vi "Simple Add.vi"() -> ()   [LabVIEW 2018]
panel:
  out "result":dbl
  in  "value 3":dbl
  in  "value 2":dbl
  in  "value":dbl
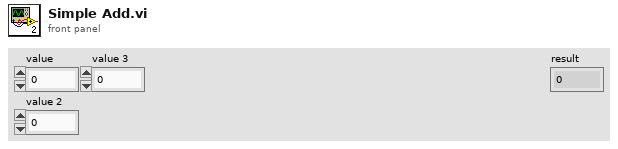
[diagram p1: front panel]
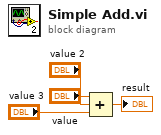
[diagram p0: block diagram]
diagram:
  n1 = Compound Arithmetic op=ADD("value", "value 2", "value 3") -> (→"result":dbl)
